vi "Image List--constant.vi"() -> (3 "image-list":path)   [LabVIEW 2021, in "TSC Button Editor.lvclass"]
doc: "This constant VI defines the location of the image list.\n\n<b>Code Developed By:</b>\nTechnology Service Corporation\nwww.tsc.com/atcs\n\nDeveloper:\nDaniel Coons"
uses:
  TSC Button Editor.lvclass
  TSC Button Editor.lvclass/TSC Button Editor.ctl
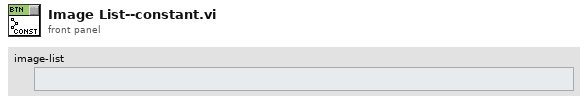
[diagram p1: front panel]
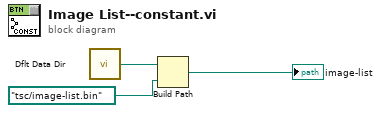
[diagram p0: block diagram]
diagram:
  n1 = call <vilib>:"Dflt Data Dir.vi"() -> ("App:Default Data Directory"=w1:path)
  n2 = Build Path(base path=w1, name or relative path=path "tsc/image-list.bin") -> (appended path=→"image-list":path)
